vi "Solve PnP (Iterative Guess).vi"(6 "Camera Parameters":T7, 8 "error in (no error)":errorcluster, 9 "Extrinsic Guess":T1, 11 "Point Correspondence Set":T4) -> (0 "error out":errorcluster, 3 "Pose":T1)   [LabVIEW 2020, in "ar.lvlib"]
doc: "Pose estimation and refinement using non-linear Levenberg-Marquardt minimization scheme."
uses:
  ar.lvlib
  common/Camera Parameters.ctl
  common/Camera Matrix.ctl
  common/Camera Distortion Coefficients.ctl
  Pose.ctl
  rvec.ctl
  tvec.ctl
  Point Correspondence Set.ctl
  common/Object Point (Float).ctl
  common/Image Point (Float).ctl
  SolvePnPFlags.ctl
  <vilib>/Utility/error.llb/Error Cluster From Error Code.vi
  common/common.lvlib
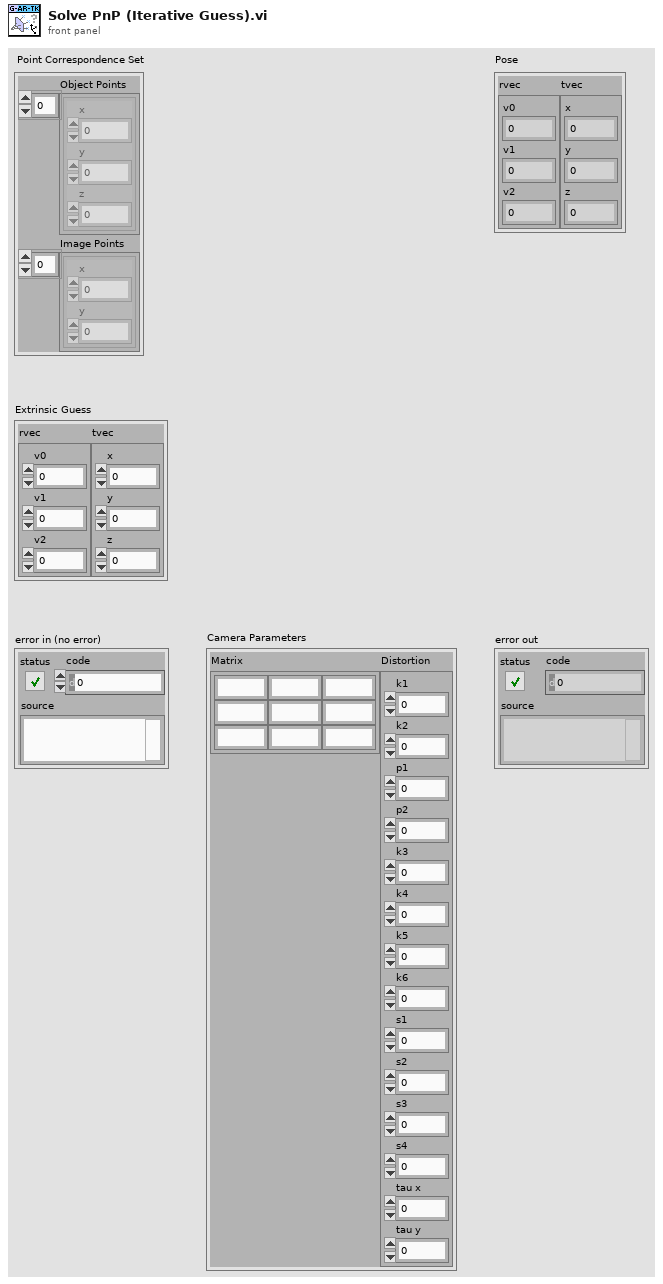
[diagram p1: front panel]
types:
  T1 = typedef "ar.lvlib/Pose.ctl" = cluster{"rvec":T2, "tvec":T3}
  T2 = typedef "ar.lvlib/rvec.ctl" = cluster{"v0":dbl, "v1":dbl, "v2":dbl}
  T3 = typedef "ar.lvlib/tvec.ctl" = cluster{"x":dbl, "y":dbl, "z":dbl}
  T4 = typedef "ar.lvlib/Point Correspondence Set.ctl" = cluster{"Object Points":T5[], "Image Points":T6[]}
  T5 = typedef "common.lvlib/Object Point (Float).ctl" = cluster{"x":dbl, "y":dbl, "z":dbl}
  T6 = typedef "common.lvlib/Image Point (Float).ctl" = cluster{"x":dbl, "y":dbl}
  T7 = typedef "common.lvlib/Camera Parameters.ctl" = cluster{"Matrix":T8, "Distortion":T9}
  T8 = typedef "common.lvlib/Camera Matrix.ctl" = cluster{"m 0,0":dbl, "m 0,1":dbl, "m 0,2":dbl, "m 1,0":dbl, "m 1,1":dbl, "m 1,2":dbl, "m 2,0":dbl, "m 2,1":dbl, "m 2,2":dbl}
  T9 = typedef "common.lvlib/Camera Distortion Coefficients.ctl" = cluster{"k1":dbl, "k2":dbl, "p1":dbl, "p2":dbl, "k3":dbl, "k4":dbl, "k5":dbl, "k6":dbl, "s1":dbl, "s2":dbl, "s3":dbl, "s4":dbl, "tau x":dbl, "tau y":dbl}
  T10 = typedef "ar.lvlib/SolvePnPFlags.ctl" = enum8{"SOLVEPNP_ITERATIVE", "SOLVEPNP_EPNP", "SOLVEPNP_P3P", "SOLVEPNP_AP3P", "SOLVEPNP_IPPE", "SOLVEPNP_IPPE_SQUARE", "SOLVEPNP_SQPNP"}
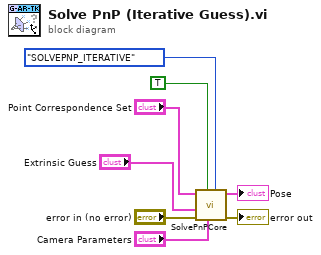
[diagram p0: block diagram]
diagram:
  n1 = call "SolvePnPCore.vi"("Solve PnP Flags"=SolvePnPFlags."SOLVEPNP_ITERATIVE", "Camera Parameters"="Camera Parameters", "Use Pose Guess"=TRUE ("Use Iterative"), "error in (no error)"="error in (no error)", "Pose (Estimate) in"="Extrinsic Guess", "Point Correspondence Set"="Point Correspondence Set") -> ("error out"=→"error out":errorcluster, "Pose"=→"Pose":T1)  [unwired: 4 in]
